vi "Execute-sequences.vi"(8 "error in (no error)":errorcluster, 11 "Object ref in":T1) -> (0 "error out":errorcluster, 3 "Object ref out":T1)   [LabVIEW 2013, in "PowderDeposition.lvlib" / "PD-Main.lvclass"]
uses:
  PD-Main.lvclass
  Object-reference.ctl
  PD-Main.lvclass/PD-Main.ctl
  Read Motor assembly.vi
  Read Abort.vi
  Read Activity log.vi
  Assembly/Motor-assembly.lvclass
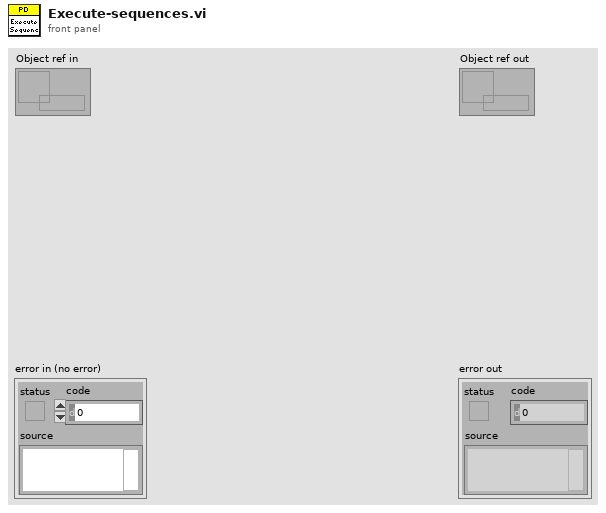
[diagram p1: front panel]
types:
  T1 = typedef "PowderDeposition.lvlib/PD-Main.lvclass/Object-reference.ctl" = refnum<data-value>
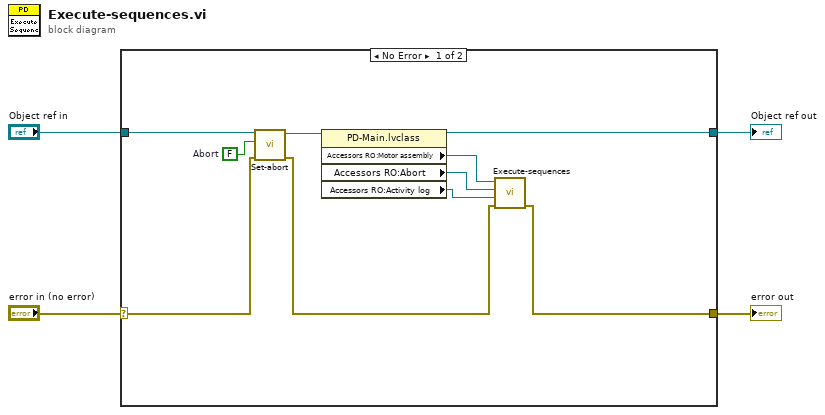
[diagram p0: block diagram]
diagram:
  n1 = case shown="No Error" "error in (no error)" {
    selector: "error in (no error)" -> [w6 w16]
    tunnel: [w11 w16] -> w3
    tunnel: [w10 w15] -> w1
    tunnel: "Object ref in" -> [w8 w15]
    frame No Error {
      w9 = FALSE  # Abort
      n2 = call "Set-abort.vi"("error in (no error)"=w6, "Abort"=w9, "Object ref in"=w8) -> ("error out"=w5:errorcluster, "Object ref out"=w7:T1)  [unwired: 7 in]
      n3 = property class="PD-Main.lvclass"(reference=w7) -> (reference out=w10:T1, "Accessors RO:Motor assembly"=w14:refnum<class "Motor-assembly.lvclass">, "Accessors RO:Abort"=w13:refnum<notifier>, "Accessors RO:Activity log"=w12:refnum<user-event>)  [unwired: 1 in, 1 out]
      n4 = call "Execute-sequences.vi"("error in (no error)"=w5, "Activity log"=w12, "Abort"=w13, "Available motors in"=w14) -> ("error out"=w11:errorcluster)  [unwired: 6 in, 1 out]
    }
    frame Error {
    }
  }
  "error out" <- w3
  "Object ref out" <- w1
